vi "Display Item.vi"(8 "error in (no error)":errorcluster, 10 "Item Panel":refnum<vi>, 11 "StoreUI in":refnum<class "StoreUI.lvclass">) -> (0 "error out":errorcluster, 3 "StoreUI out":refnum<class "StoreUI.lvclass">)   [LabVIEW 2015, in "StoreUI.lvlib" / "StoreUI.lvclass"]
uses:
  StoreUI.lvclass
  StoreUI.lvclass/StoreUI.ctl
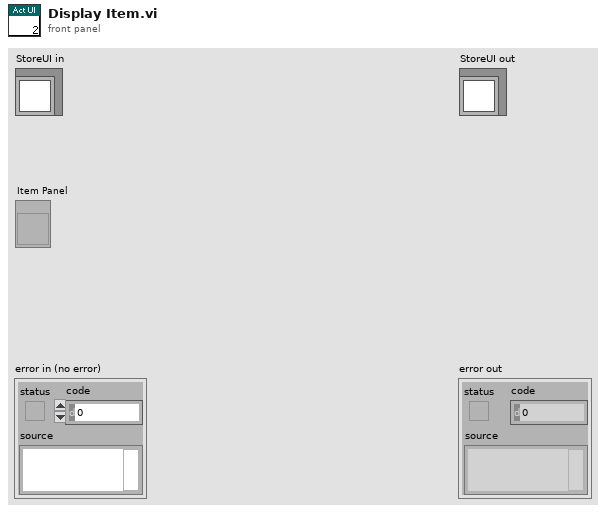
[diagram p1: front panel]
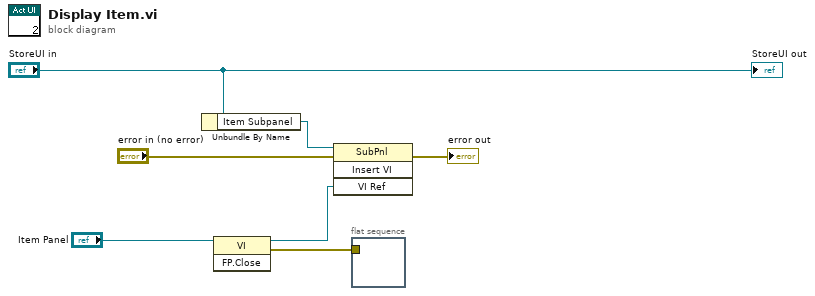
[diagram p0: block diagram]
diagram:
  n1 = Unbundle By Name("StoreUI in") -> ("Item Subpanel"=w3:refnum<vi>)
  n2 = invoke class="VI" method="FP.Close"(reference="Item Panel") -> (reference out=w2:refnum<vi>, error out=w1:errorcluster)  [unwired: 2 in, 1 out]
  n3 = invoke class="SubPnl" method="Insert VI"(reference=w3, error in="error in (no error)", "VI Ref"=w2) -> (error out=→"error out":errorcluster)  [unwired: 1 in, 3 out]
  n4 = flat-sequence {
    tunnel: w1 -> [_]
    frame #0 {
    }
  }
  "StoreUI out" <- "StoreUI in"
